vi "Get.vi"(8 "error in (no error)":errorcluster, 11 "MsgPackDeserializer in":refnum<class "MsgPackDeserializer.lvclass">) -> (0 "error out":errorcluster, 2 "Variant":variant, 3 "MsgPackDeserializer out":refnum<class "MsgPackDeserializer.lvclass">)   [LabVIEW 2015, in "MsgPackDeserializer.lvclass"]
uses:
  MsgPackDeserializer.lvclass
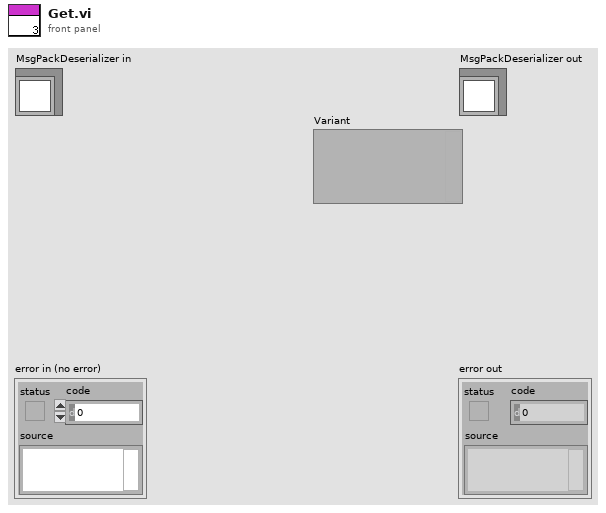
[diagram p1: front panel]
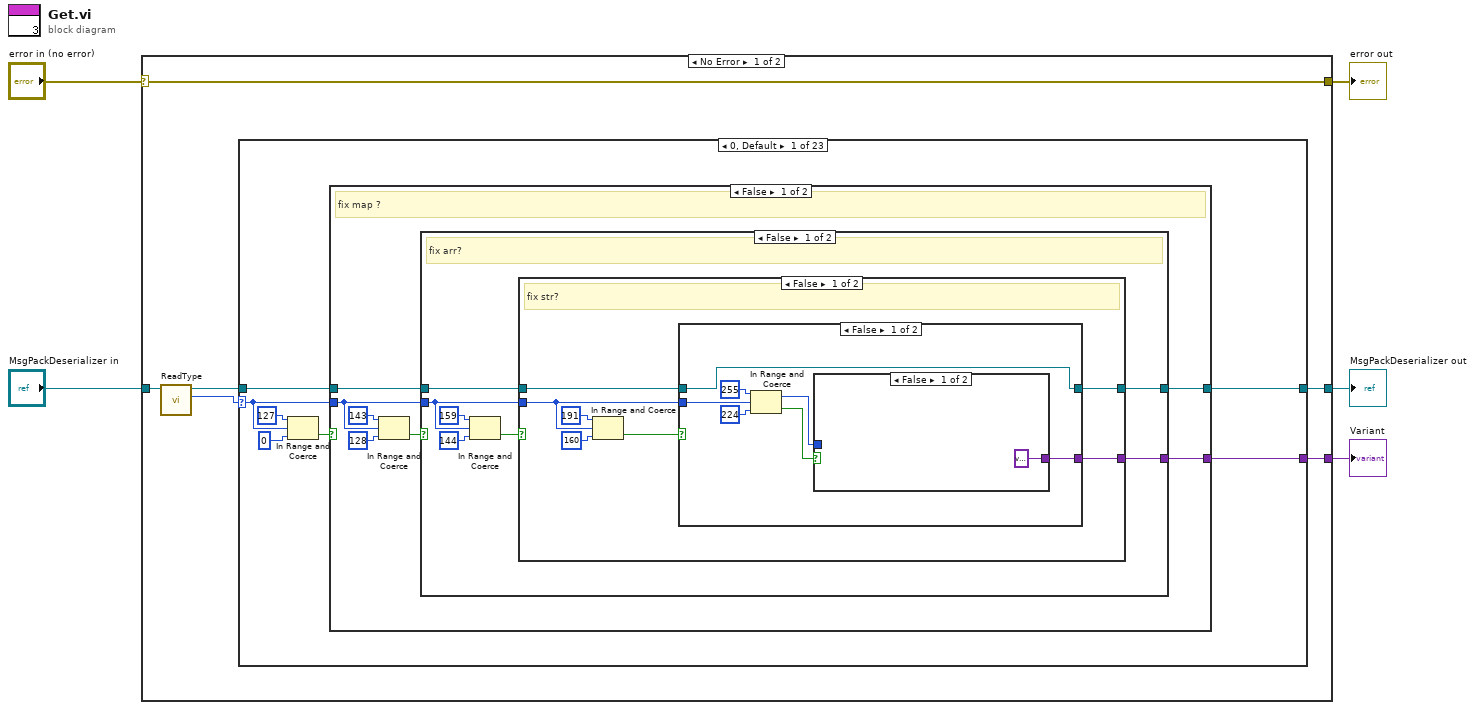
[diagram p0: block diagram]
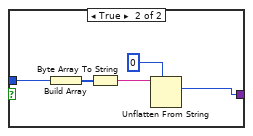
[diagram p2: hidden frame]
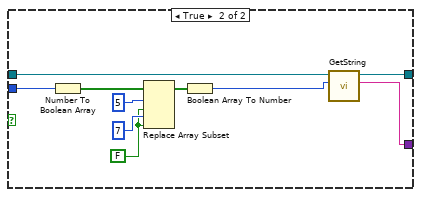
[diagram p3: hidden frame]
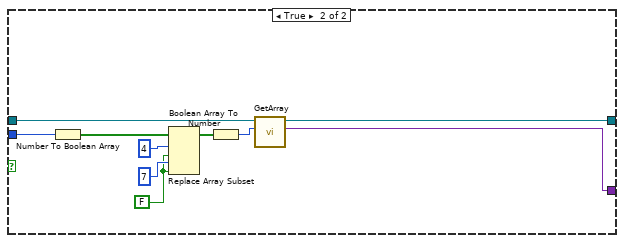
[diagram p4: hidden frame]
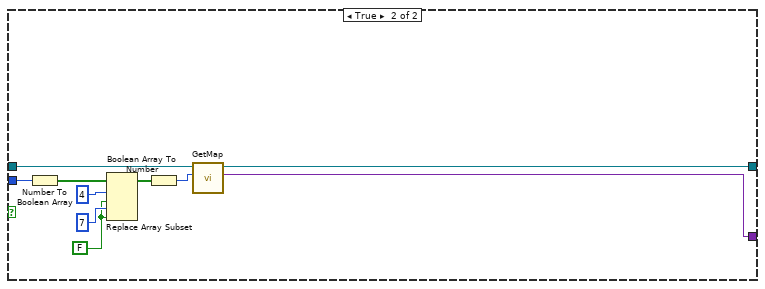
[diagram p5: hidden frame]
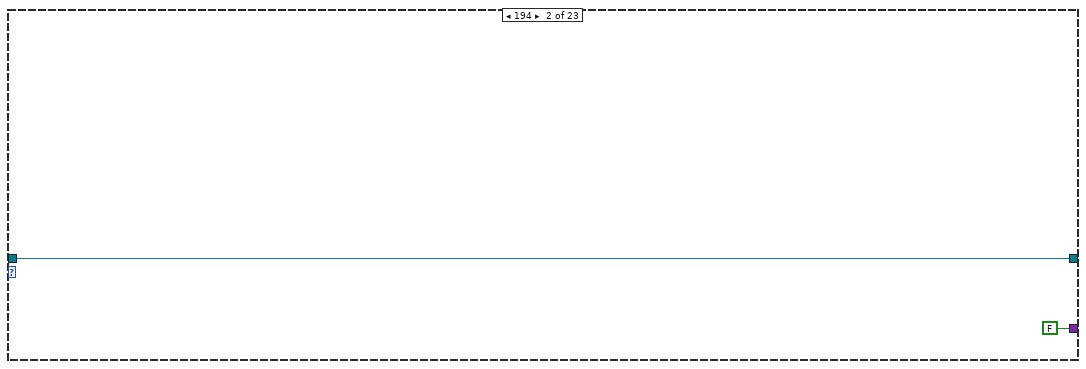
[diagram p7: hidden frame]
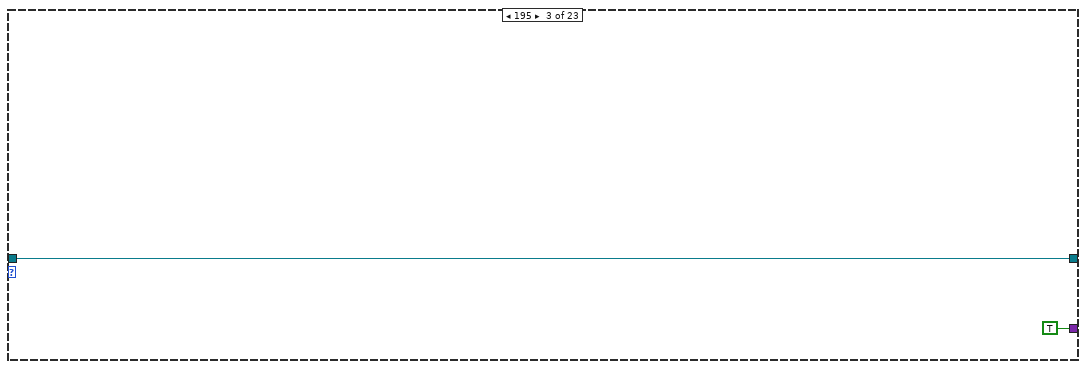
[diagram p8: hidden frame]
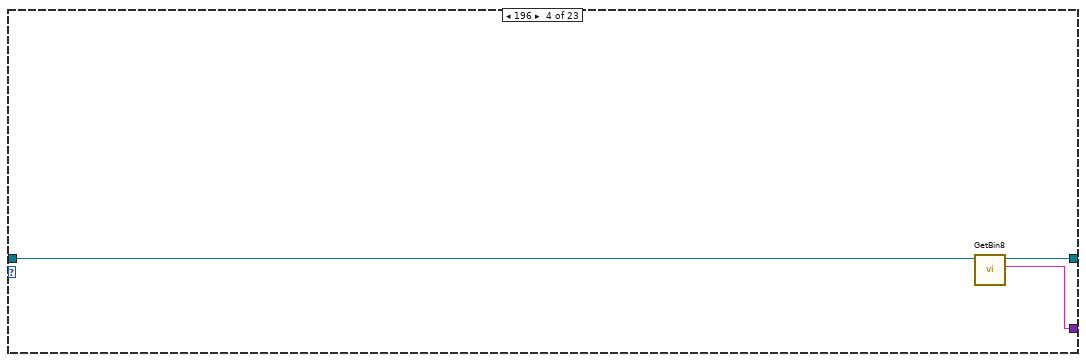
[diagram p9: hidden frame]
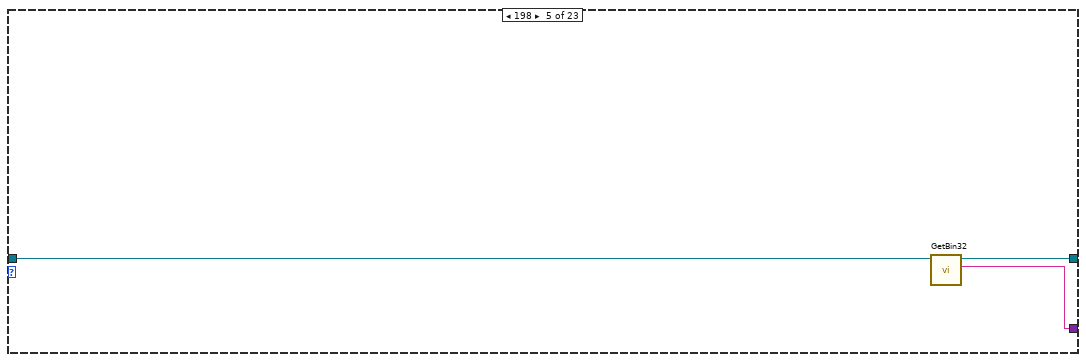
[diagram p10: hidden frame]
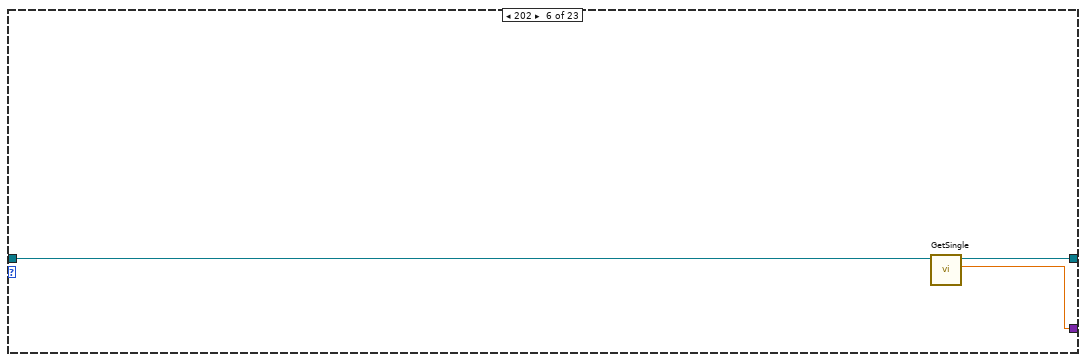
[diagram p11: hidden frame]
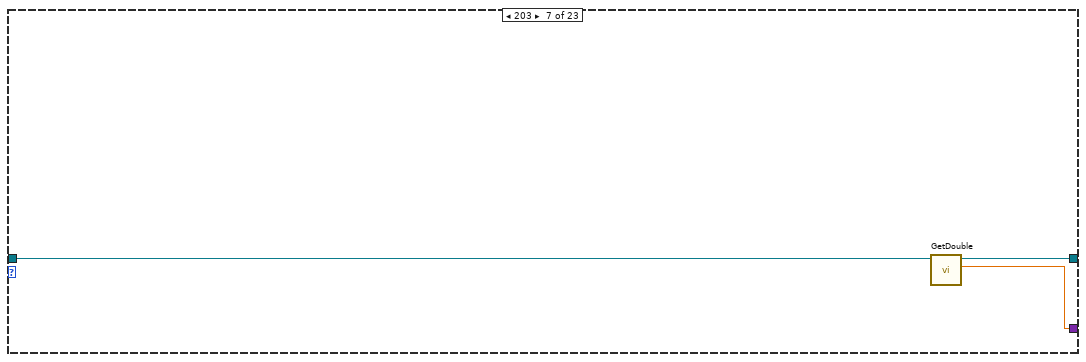
[diagram p12: hidden frame]
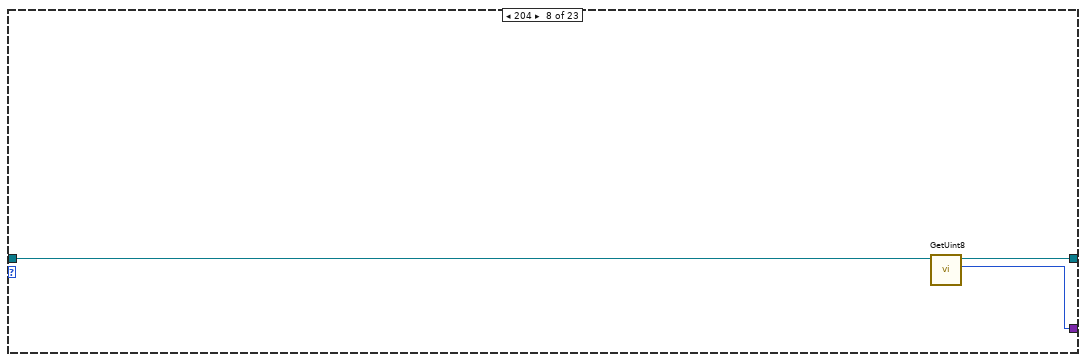
[diagram p13: hidden frame]
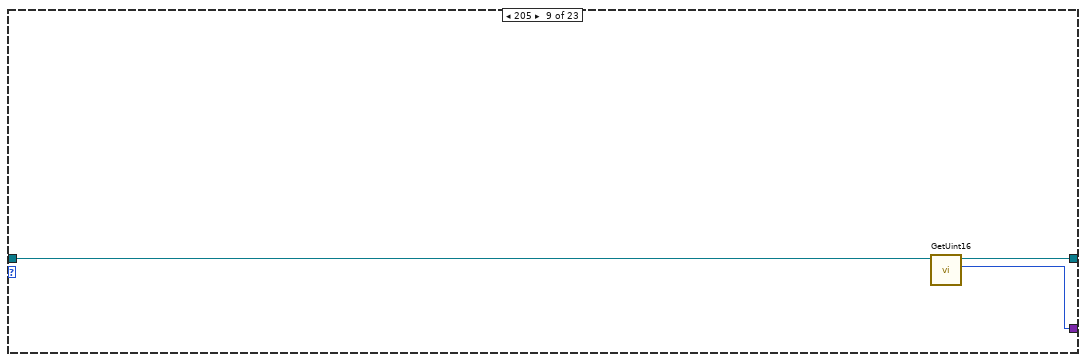
[diagram p14: hidden frame]
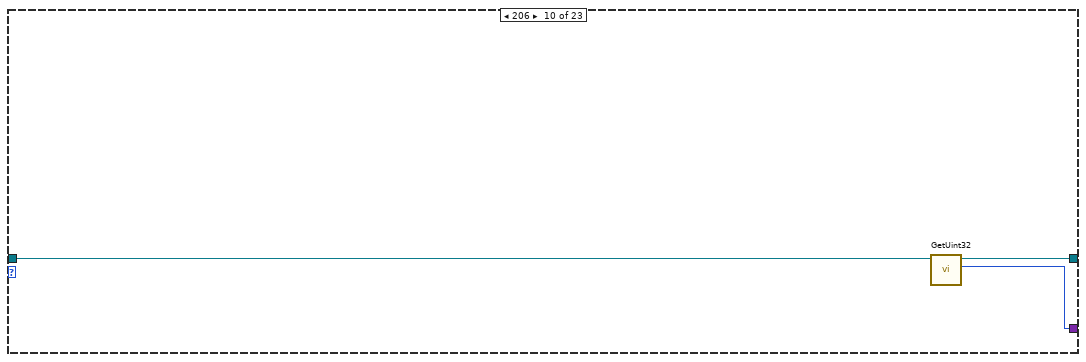
[diagram p15: hidden frame]
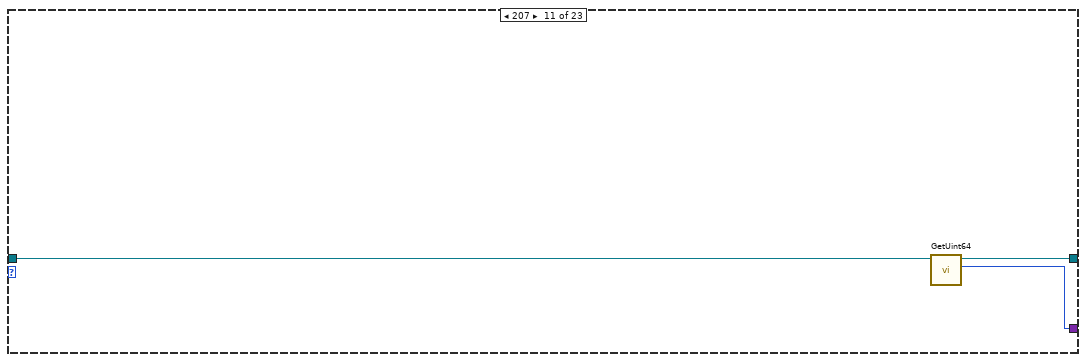
[diagram p16: hidden frame]
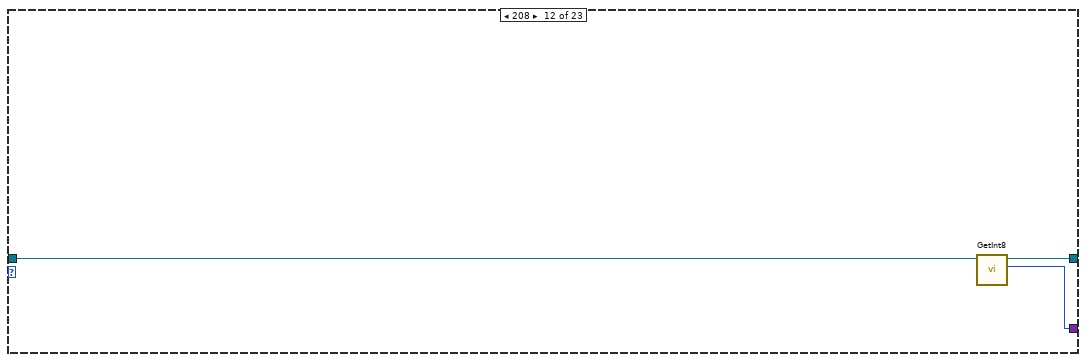
[diagram p17: hidden frame]
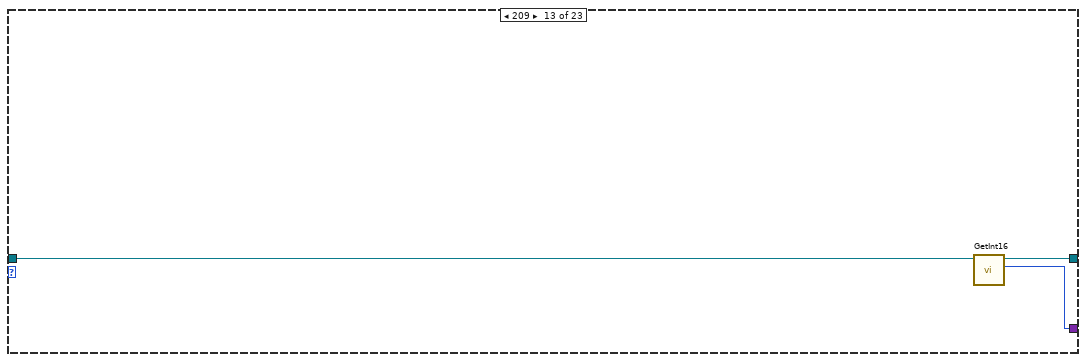
[diagram p18: hidden frame]
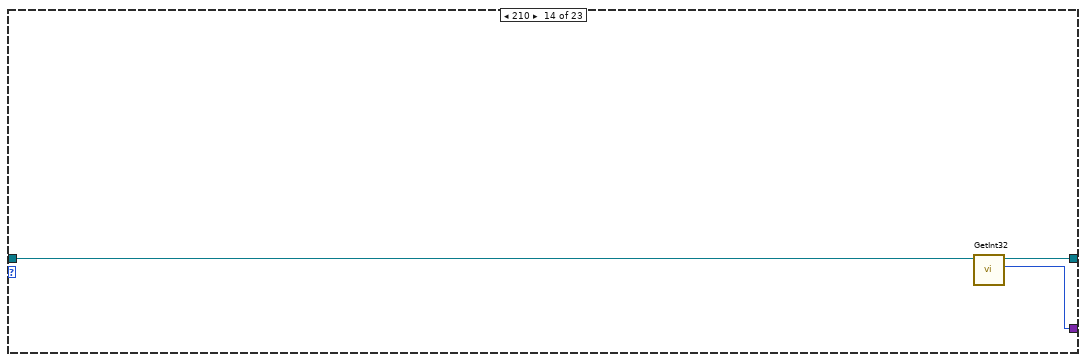
[diagram p19: hidden frame]
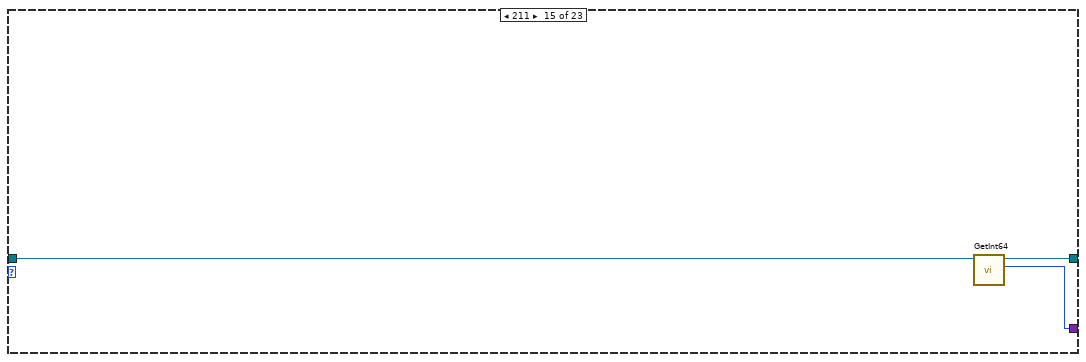
[diagram p20: hidden frame]
diagram:
  n1 = case shown="No Error" "error in (no error)" {
    selector: "error in (no error)" -> [w11 w158]
    tunnel: [w11 w158] -> w4
    tunnel: [w6 w157] -> w2
    tunnel: "MsgPackDeserializer in" -> [w10 w157]
    tunnel: [w8 _] -> w1
    frame No Error {
      n2 = call "ReadType.vi"("MsgPackDeserializer in"=w10) -> ("Type"=w9:u8, "MsgPackDeserializer out"=w7:refnum<class "MsgPackDeserializer.lvclass">)  [unwired: 8 in, 1 out]
      n3 = case shown="0, Default" w9 {
        selector: w9 -> [w14 _ _ _ _ _ _ _ _ _ _ _ _ _ _ _ _ _ _ _ _ _ _]
        tunnel: [w15 FALSE TRUE w91 w92 w95 w98 w101 w104 w108 w110 w114 w117 w120 w123 w125 w129 w132 w135 w143 w144 w149 w155] -> w8
        tunnel: w7 -> [w13 w85 w87 w90 w94 w97 w100 w103 w106 w109 w112 w115 w118 w121 w124 w127 w130 w133 w138 w141 w148 w153 w156]
        tunnel: [w12 w85 w87 w89 w93 w96 w99 w102 w105 w107 w111 w113 w116 w119 w122 w126 w128 w131 w134 w142 w145 w150 w154] -> w6
        frame 0, Default {
          n4 = In Range and Coerce(upper limit=u8 127, x=w14, lower limit=u8 0 ("upper limit")) -> (In Range?=w16:bool)  [unwired: 1 out]
          n5 = case shown="False" w16 {
            tunnel: [w22 w84] -> w15
            tunnel: w14 -> [w21 w84]
            tunnel: w13 -> [w20 w83]
            tunnel: [w19 w83] -> w12
            frame False {
              # "fix map ?"
              n6 = In Range and Coerce(upper limit=u8 143, x=w21, lower limit=u8 128 ("upper limit")) -> (In Range?=w23:bool)  [unwired: 1 out]
              n7 = case shown="False" w23 {
                tunnel: [w26 w74] -> w22
                tunnel: w21 -> [w29 w77]
                tunnel: w20 -> [w28 w76]
                tunnel: [w27 w75] -> w19
                frame False {
                  # "fix arr?"
                  n8 = In Range and Coerce(upper limit=u8 159, x=w29, lower limit=u8 144 ("upper limit")) -> (In Range?=w30:bool)  [unwired: 1 out]
                  n9 = case shown="False" w30 {
                    tunnel: w29 -> [w37 w67]
                    tunnel: w28 -> [w35 w66]
                    tunnel: [w34 w63] -> w27
                    tunnel: [w33 w64] -> w26
                    frame False {
                      # "fix str?"
                      n10 = In Range and Coerce(upper limit=u8 191, x=w37, lower limit=u8 160 ("upper limit")) -> (In Range?=w36:bool)  [unwired: 1 out]
                      n11 = case shown="False" w36 {
                        tunnel: w37 -> [w43 w62]
                        tunnel: w35 -> [w46 w56]
                        tunnel: [w46 w55] -> w34
                        tunnel: [w40 w53] -> w33
                        frame False {
                          n12 = In Range and Coerce(upper limit=u8 255, x=w43, lower limit=u8 224 ("upper limit")) -> (coerced(x)=w42:u8, In Range?=w41:bool)
                          n13 = case shown="False" w41 {
                            tunnel: w42 -> [_ w52]
                            tunnel: [variant ("Variant") w48] -> w40
                            frame False {
                            }
                            frame True {
                              n14 = Build Array(w52) -> (w50:u8[])
                              n15 = Byte Array To String(unsigned byte array=w50) -> (string=w51:string)
                              n16 = Unflatten From String(type=i8 0 ("upper limit"), binary string=w51) -> (value=w48:i8)  [unwired: 3 in, 2 out]
                            }
                          }
                        }
                        frame True {
                          w57 = FALSE ("new element/subarray")
                          n17 = Number To Boolean Array(number=w62) -> (Boolean array=w61:bool[])
                          n18 = Replace Array Subset(array=w61, new element #1=w57, index #1=5 ("index"), new element #2=w57, index #2=7 ("index")) -> (w59:bool[])
                          n19 = Boolean Array To Number(Boolean array=w59) -> (number=w54:u32)
                          n20 = call "GetString.vi"("length"=w54, "MsgPackDeserializer in"=w56) -> ("data"=w53:string, "MsgPackDeserializer out"=w55:refnum<class "MsgPackDeserializer.lvclass">)  [unwired: 7 in, 1 out]
                        }
                      }
                    }
                    frame True {
                      w69 = FALSE ("new element/subarray")
                      n21 = Number To Boolean Array(number=w67) -> (Boolean array=w68:bool[])
                      n22 = Replace Array Subset(array=w68, new element #1=w69, index #1=4 ("index"), new element #2=w69, index #2=7 ("index")) -> (w71:bool[])
                      n23 = Boolean Array To Number(Boolean array=w71) -> (number=w65:u32)
                      n24 = call "GetArray.vi"("size"=w65, "MsgPackDeserializer in"=w66) -> ("Variant"=w64:variant, "MsgPackDeserializer out"=w63:refnum<class "MsgPackDeserializer.lvclass">)  [unwired: 7 in, 1 out]
                    }
                  }
                }
                frame True {
                  w79 = FALSE ("new element/subarray")
                  n25 = Number To Boolean Array(number=w77) -> (Boolean array=w78:bool[])
                  n26 = Replace Array Subset(array=w78, new element #1=w79, index #1=4 ("index"), new element #2=w79, index #2=7 ("index")) -> (w81:bool[])
                  n27 = Boolean Array To Number(Boolean array=w81) -> (number=w73:u32)
                  n28 = call "GetMap.vi"("size"=w73, "MsgPackDeserializer in"=w76) -> ("Variant"=w74:variant, "MsgPackDeserializer out"=w75:refnum<class "MsgPackDeserializer.lvclass">)  [unwired: 7 in, 1 out]
                }
              }
            }
            frame True {
              # "fix pos"
            }
          }
        }
        frame 194 {
        }
        frame 195 {
        }
        frame 196 {
          n29 = call "GetBin8.vi"("MsgPackDeserializer in"=w90) -> ("data"=w91:string, "MsgPackDeserializer out"=w89:refnum<class "MsgPackDeserializer.lvclass">)  [unwired: 8 in, 1 out]
        }
        frame 198 {
          n30 = call "GetBin32.vi"("MsgPackDeserializer in"=w94) -> ("data"=w92:string, "MsgPackDeserializer out"=w93:refnum<class "MsgPackDeserializer.lvclass">)  [unwired: 8 in, 1 out]
        }
        frame 202 {
          n31 = call "GetSingle.vi"("MsgPackDeserializer in"=w97) -> ("Number"=w95:sgl, "MsgPackDeserializer out"=w96:refnum<class "MsgPackDeserializer.lvclass">)  [unwired: 8 in, 1 out]
        }
        frame 203 {
          n32 = call "GetDouble.vi"("MsgPackDeserializer in"=w100) -> ("Number"=w98:dbl, "MsgPackDeserializer out"=w99:refnum<class "MsgPackDeserializer.lvclass">)  [unwired: 8 in, 1 out]
        }
        frame 204 {
          n33 = call "GetUint8.vi"("MsgPackDeserializer in"=w103) -> ("Number"=w101:u8, "MsgPackDeserializer out"=w102:refnum<class "MsgPackDeserializer.lvclass">)  [unwired: 8 in, 1 out]
        }
        frame 205 {
          n34 = call "GetUint16.vi"("MsgPackDeserializer in"=w106) -> ("Number"=w104:u16, "MsgPackDeserializer out"=w105:refnum<class "MsgPackDeserializer.lvclass">)  [unwired: 8 in, 1 out]
        }
        frame 206 {
          n35 = call "GetUint32.vi"("MsgPackDeserializer in"=w109) -> ("Number"=w108:u32, "MsgPackDeserializer out"=w107:refnum<class "MsgPackDeserializer.lvclass">)  [unwired: 8 in, 1 out]
        }
        frame 207 {
          n36 = call "GetUint64.vi"("MsgPackDeserializer in"=w112) -> ("Number"=w110:u64, "MsgPackDeserializer out"=w111:refnum<class "MsgPackDeserializer.lvclass">)  [unwired: 8 in, 1 out]
        }
        frame 208 {
          n37 = call "GetInt8.vi"("MsgPackDeserializer in"=w115) -> ("Number"=w114:i8, "MsgPackDeserializer out"=w113:refnum<class "MsgPackDeserializer.lvclass">)  [unwired: 8 in, 1 out]
        }
        frame 209 {
          n38 = call "GetInt16.vi"("MsgPackDeserializer in"=w118) -> ("Number"=w117:i16, "MsgPackDeserializer out"=w116:refnum<class "MsgPackDeserializer.lvclass">)  [unwired: 8 in, 1 out]
        }
        frame 210 {
          n39 = call "GetInt32.vi"("MsgPackDeserializer in"=w121) -> ("Number"=w120:i32, "MsgPackDeserializer out"=w119:refnum<class "MsgPackDeserializer.lvclass">)  [unwired: 8 in, 1 out]
        }
        frame 211 {
          n40 = call "GetInt64.vi"("MsgPackDeserializer in"=w124) -> ("Number"=w123:i64, "MsgPackDeserializer out"=w122:refnum<class "MsgPackDeserializer.lvclass">)  [unwired: 8 in, 1 out]
        }
        frame 217 {
          n41 = call "GetBin8.vi"("MsgPackDeserializer in"=w127) -> ("data"=w125:string, "MsgPackDeserializer out"=w126:refnum<class "MsgPackDeserializer.lvclass">)  [unwired: 8 in, 1 out]
        }
        frame 218 {
          n42 = call "GetBin16.vi"("MsgPackDeserializer in"=w130) -> ("data"=w129:string, "MsgPackDeserializer out"=w128:refnum<class "MsgPackDeserializer.lvclass">)  [unwired: 8 in, 1 out]
        }
        frame 219 {
          n43 = call "GetBin32.vi"("MsgPackDeserializer in"=w133) -> ("data"=w132:string, "MsgPackDeserializer out"=w131:refnum<class "MsgPackDeserializer.lvclass">)  [unwired: 8 in, 1 out]
        }
        frame 220 {
          n44 = call "GetUint16.vi"("MsgPackDeserializer in"=w138) -> ("Number"=w137:u16, "MsgPackDeserializer out"=w136:refnum<class "MsgPackDeserializer.lvclass">)  [unwired: 8 in, 1 out]
          n45 = call "GetArray.vi"("size"=w137, "MsgPackDeserializer in"=w136) -> ("Variant"=w135:variant, "MsgPackDeserializer out"=w134:refnum<class "MsgPackDeserializer.lvclass">)  [unwired: 7 in, 1 out]
        }
        frame 221 {
          n46 = call "GetUint32.vi"("MsgPackDeserializer in"=w141) -> ("Number"=w139:u32, "MsgPackDeserializer out"=w140:refnum<class "MsgPackDeserializer.lvclass">)  [unwired: 8 in, 1 out]
          n47 = call "GetArray.vi"("size"=w139, "MsgPackDeserializer in"=w140) -> ("Variant"=w143:variant, "MsgPackDeserializer out"=w142:refnum<class "MsgPackDeserializer.lvclass">)  [unwired: 7 in, 1 out]
        }
        frame 222 {
          n48 = call "GetUint16.vi"("MsgPackDeserializer in"=w148) -> ("Number"=w147:u16, "MsgPackDeserializer out"=w146:refnum<class "MsgPackDeserializer.lvclass">)  [unwired: 8 in, 1 out]
          n49 = call "GetMap.vi"("size"=w147, "MsgPackDeserializer in"=w146) -> ("Variant"=w144:variant, "MsgPackDeserializer out"=w145:refnum<class "MsgPackDeserializer.lvclass">)  [unwired: 7 in, 1 out]
        }
        frame 223 {
          n50 = call "GetUint32.vi"("MsgPackDeserializer in"=w153) -> ("Number"=w152:u32, "MsgPackDeserializer out"=w151:refnum<class "MsgPackDeserializer.lvclass">)  [unwired: 8 in, 1 out]
          n51 = call "GetMap.vi"("size"=w152, "MsgPackDeserializer in"=w151) -> ("Variant"=w149:variant, "MsgPackDeserializer out"=w150:refnum<class "MsgPackDeserializer.lvclass">)  [unwired: 7 in, 1 out]
        }
        frame 197 {
          n52 = call "GetBin16.vi"("MsgPackDeserializer in"=w156) -> ("data"=w155:string, "MsgPackDeserializer out"=w154:refnum<class "MsgPackDeserializer.lvclass">)  [unwired: 8 in, 1 out]
        }
      }
    }
    frame Error {
    }
  }
  "error out" <- w4
  "MsgPackDeserializer out" <- w2
  "Variant" <- w1
